vi "Formatacao de Waveform.vi"(3 "Array in":dbl[](array[numeric])) -> (0 "Tank Levels":waveform(dbl)[](array[waveform]), 1 "Pump Voltages":waveform(dbl)[](array[waveform]))   [LabVIEW 2018]
uses:
  GV Config.vi
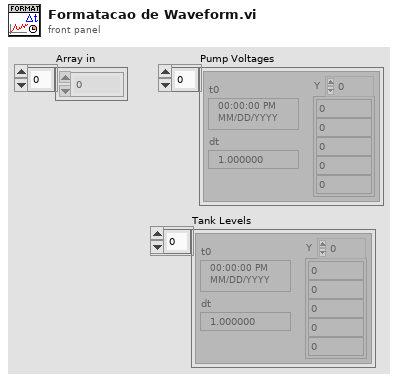
[diagram p1: front panel]
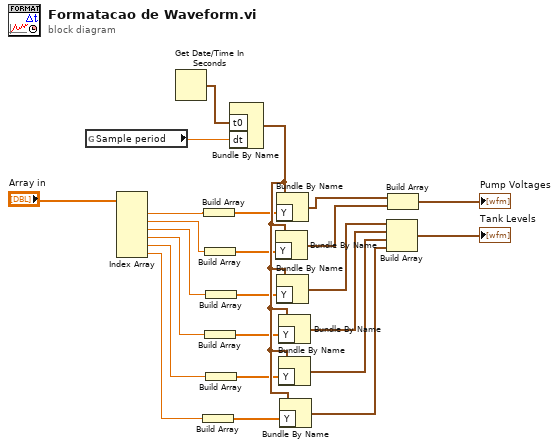
[diagram p0: block diagram]
diagram:
  n1 = global read "GV Config.vi" "Sample period"() -> (w1:dbl)
  n2 = Index Array(array="Array in") -> (element #1=w18:dbl, element #2=w16:dbl, element #3=w15:dbl, element #4=w13:dbl, element #5=w11:dbl, element #6=w9:dbl)  [unwired: 6 in]
  n3 = Get Date/Time In Seconds() -> (seconds since 1Jan1904=w22:timestamp)
  n4 = Build Array(w9) -> (w8:dbl[])
  n5 = Build Array(w18) -> (w19:dbl[])
  n6 = Build Array(w16) -> (w17:dbl[])
  n7 = Build Array(w13) -> (w12:dbl[])
  n8 = Build Array(w15) -> (w14:dbl[])
  n9 = Build Array(w11) -> (w10:dbl[])
  n10 = Bundle By Name("t0"=w22, "dt"=w1) -> (w20:waveform(dbl))  [unwired: 1 in]
  n11 = Bundle By Name(cluster=w20, "Y"=w17) -> (w5:waveform(dbl))
  n12 = Bundle By Name(cluster=w20, "Y"=w19) -> (w4:waveform(dbl))
  n13 = Bundle By Name(cluster=w20, "Y"=w14) -> (w24:waveform(dbl))
  n14 = Bundle By Name(cluster=w20, "Y"=w12) -> (w21:waveform(dbl))
  n15 = Bundle By Name(cluster=w20, "Y"=w10) -> (w7:waveform(dbl))
  n16 = Bundle By Name(cluster=w20, "Y"=w8) -> (w6:waveform(dbl))
  n17 = Build Array(w24, w21, w7, w6) -> (→"Tank Levels":waveform(dbl)[])
  n18 = Build Array(w4, w5) -> (→"Pump Voltages":waveform(dbl)[])
